vi "UserPrompt__slk_mt.vi"(8 "error in (no error)":errorcluster, 11 "new frame name in (\"\")":string) -> (0 "error out":errorcluster, 2 "ok?":bool, 3 "new frame name out":string)   [LabVIEW 2015, in "Lazyboots Menu Tool.lvlib"]
uses:
  <vilib>/SLK/Lazyboots Menu Tool/Library/Lazyboots Menu Tool.lvlib
panel:
  in  "cancel":bool
  in  "ok":bool
  in  "new frame name":string caption="New Frame Name:"
  # "Please input new frame name here then press \"OK\" or press \"Cancel\"."
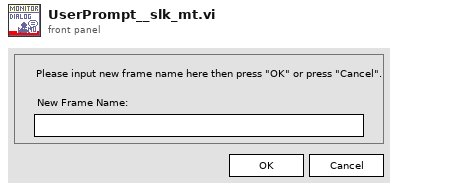
[diagram p1: front panel]
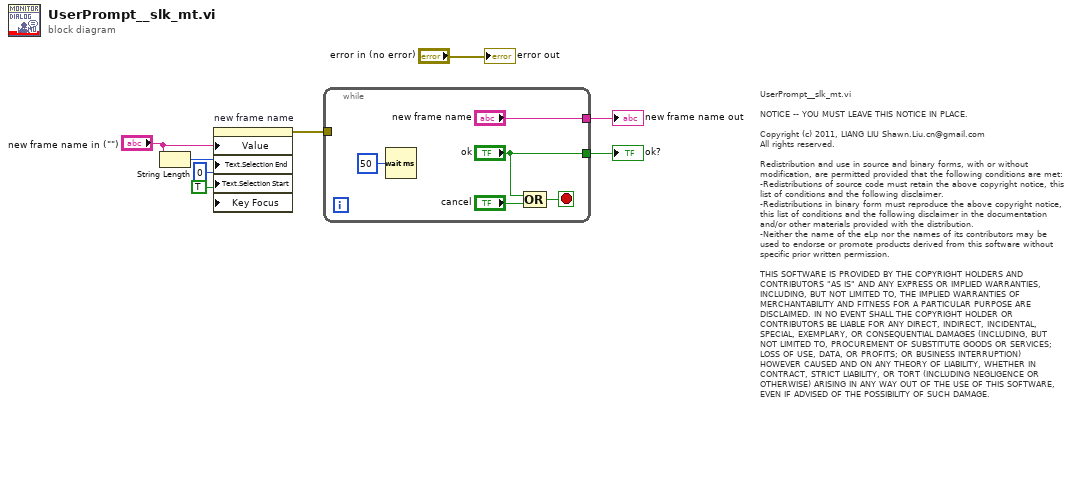
[diagram p0: block diagram]
diagram:
  # "UserPrompt__slk_mt.vi\n\nNOTICE -- YOU MUST LEAVE THIS NOTICE IN PLACE.\n\nCopyright (c) 2011, LIANG LIU Shawn.Liu.cn@gmail.com\nAll rights reserved.\n\nRedistribution and use in source and binary forms, with or without modification, are permitted provided that the following conditions are met:\n-Redistributions of source code must retain the above copyright notice, this list of conditions and the following disclaimer.\n-Redistributions in binary form must reproduce the above copyright notice, this list of conditions and the following disclaimer in the documentation and/or other materials provided with the distribution.\n-Neither the name of the eLp nor the names of its contributors may be used to endorse or promote products derived from this software without specific prior written permission.\n\nTHIS SOFTWARE IS PROVIDED BY THE COPYRIGHT HOLDERS AND CONTRIBUTORS \"AS IS\" AND ANY EXPRESS OR IMPLIED WARRANTIES, INCLUDING, BUT NOT LIMITED TO, THE IMPLIED WARRANTIES OF MERCHANTABILITY AND FITNESS FOR A PARTICULAR PURPOSE ARE DISCLAIMED. IN NO EVENT SHALL THE COPYRIGHT HOLDER OR CONTRIBUTORS BE LIABLE FOR ANY DIRECT, INDIRECT, INCIDENTAL, SPECIAL, EXEMPLARY, OR CONSEQUENTIAL DAMAGES (INCLUDING, BUT NOT LIMITED TO, PROCUREMENT OF SUBSTITUTE GOODS OR SERVICES; LOSS OF USE, DATA, OR PROFITS; OR BUSINESS INTERRUPTION) HOWEVER CAUSED AND ON ANY THEORY OF LIABILITY, WHETHER IN CONTRACT, STRICT LIABILITY, OR TORT (INCLUDING NEGLIGENCE OR OTHERWISE) ARISING IN ANY WAY OUT OF THE USE OF THIS SOFTWARE, EVEN IF ADVISED OF THE POSSIBILITY OF SUCH DAMAGE."
  n1 = String Length(string="new frame name in (\"\")") -> (length=w4:i32)
  n2 = property on="new frame name" class="Str"("Value"="new frame name in (\"\")", "Text.Selection End"=w4, "Text.Selection Start"=u32 0 ("Text.Selection:Start"), "Key Focus"=TRUE) -> (error out=w5:errorcluster)  [unwired: 2 in, 1 out]
  n3 = while {
    tunnel: ["new frame name"] -> w7
    tunnel: ["ok"] -> w6
    tunnel: w5 -> [_]
    stop <- w11 stop-if-true
    n4 = Wait (ms)(milliseconds to wait=u32 50) -> ()  [unwired: 1 out]
    n5 = Compound Arithmetic op=OR("ok", "cancel") -> (w11:bool)
  }
  "ok?" <- w6
  "new frame name out" <- w7
  "error out" <- "error in (no error)"
